vi "Parallel_FFTs.vi"(10 "SampleRate":dbl, 11 "Y":cdb[](array[numeric])) -> (2 "PeakValues":dbl[](array[numeric]), 3 "10 Hz FFTs":dbl[][](array[numeric]))   [LabVIEW 2018]
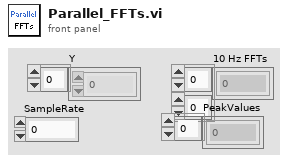
[diagram p1: front panel]
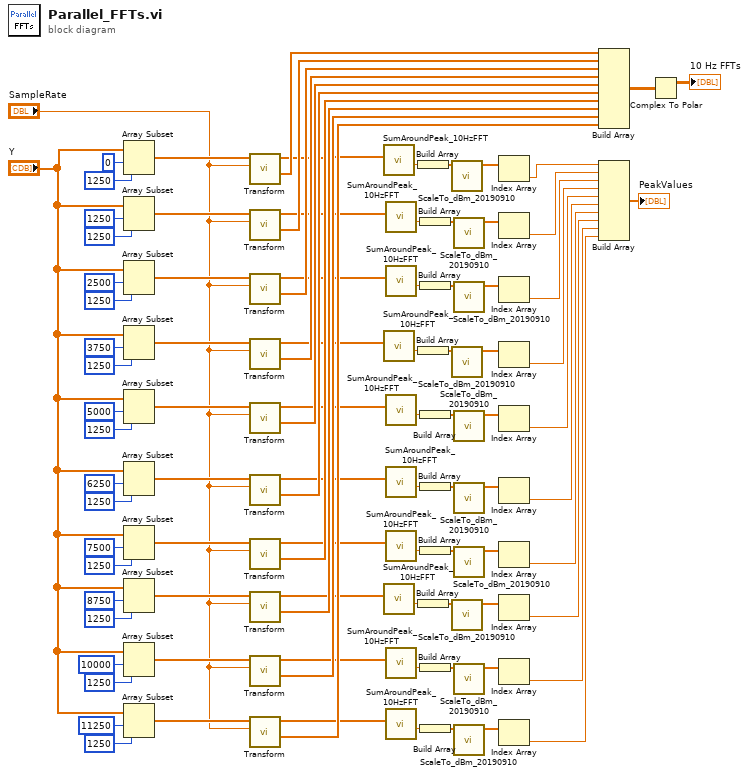
[diagram p0: block diagram]
diagram:
  n1 = Array Subset(array="Y", index=0, length=1250) -> (w76:cdb[])
  n2 = Array Subset(array="Y", index=1250, length=1250) -> (w77:cdb[])
  n3 = Array Subset(array="Y", index=2500, length=1250) -> (w78:cdb[])
  n4 = Array Subset(array="Y", index=3750, length=1250) -> (w79:cdb[])
  n5 = Array Subset(array="Y", index=5000, length=1250) -> (w80:cdb[])
  n6 = Array Subset(array="Y", index=6250, length=1250) -> (w81:cdb[])
  n7 = Array Subset(array="Y", index=7500, length=1250) -> (w82:cdb[])
  n8 = Array Subset(array="Y", index=8750, length=1250) -> (w83:cdb[])
  n9 = Array Subset(array="Y", index=10000, length=1250) -> (w84:cdb[])
  n10 = Array Subset(array="Y", index=11250, length=1250) -> (w85:cdb[])
  n11 = call "Transform.vi"("SampleRate"="SampleRate", "TimeDomainIn"=w76) -> ("Complex"=w61:cdb[], "AmplitudeSpectrum"=w44:dbl[])  [unwired: 4 in, 4 out]
  n12 = call "Transform.vi"("SampleRate"="SampleRate", "TimeDomainIn"=w77) -> ("Complex"=w60:cdb[], "AmplitudeSpectrum"=w49:dbl[])  [unwired: 4 in, 4 out]
  n13 = call "Transform.vi"("SampleRate"="SampleRate", "TimeDomainIn"=w78) -> ("Complex"=w59:cdb[], "AmplitudeSpectrum"=w41:dbl[])  [unwired: 4 in, 4 out]
  n14 = call "Transform.vi"("SampleRate"="SampleRate", "TimeDomainIn"=w79) -> ("Complex"=w58:cdb[], "AmplitudeSpectrum"=w32:dbl[])  [unwired: 4 in, 4 out]
  n15 = call "Transform.vi"("SampleRate"="SampleRate", "TimeDomainIn"=w80) -> ("Complex"=w57:cdb[], "AmplitudeSpectrum"=w33:dbl[])  [unwired: 4 in, 4 out]
  n16 = call "Transform.vi"("SampleRate"="SampleRate", "TimeDomainIn"=w81) -> ("Complex"=w56:cdb[], "AmplitudeSpectrum"=w34:dbl[])  [unwired: 4 in, 4 out]
  n17 = call "Transform.vi"("SampleRate"="SampleRate", "TimeDomainIn"=w82) -> ("Complex"=w55:cdb[], "AmplitudeSpectrum"=w23:dbl[])  [unwired: 4 in, 4 out]
  n18 = call "Transform.vi"("SampleRate"="SampleRate", "TimeDomainIn"=w83) -> ("Complex"=w54:cdb[], "AmplitudeSpectrum"=w22:dbl[])  [unwired: 4 in, 4 out]
  n19 = call "Transform.vi"("SampleRate"="SampleRate", "TimeDomainIn"=w84) -> ("Complex"=w53:cdb[], "AmplitudeSpectrum"=w21:dbl[])  [unwired: 4 in, 4 out]
  n20 = call "Transform.vi"("SampleRate"="SampleRate", "TimeDomainIn"=w85) -> ("Complex"=w52:cdb[], "AmplitudeSpectrum"=w20:dbl[])  [unwired: 4 in, 4 out]
  n21 = call "SumAroundPeak_10HzFFT.vi"("spectrum in"=w44) -> ("SumOfPeak"=w46:dbl)  [unwired: 8 in, 2 out]
  n22 = call "SumAroundPeak_10HzFFT.vi"("spectrum in"=w32) -> ("SumOfPeak"=w38:dbl)  [unwired: 8 in, 2 out]
  n23 = call "SumAroundPeak_10HzFFT.vi"("spectrum in"=w22) -> ("SumOfPeak"=w28:dbl)  [unwired: 8 in, 2 out]
  n24 = call "SumAroundPeak_10HzFFT.vi"("spectrum in"=w49) -> ("SumOfPeak"=w50:dbl)  [unwired: 8 in, 2 out]
  n25 = call "SumAroundPeak_10HzFFT.vi"("spectrum in"=w41) -> ("SumOfPeak"=w42:dbl)  [unwired: 8 in, 2 out]
  n26 = call "SumAroundPeak_10HzFFT.vi"("spectrum in"=w33) -> ("SumOfPeak"=w35:dbl)  [unwired: 8 in, 2 out]
  n27 = call "SumAroundPeak_10HzFFT.vi"("spectrum in"=w34) -> ("SumOfPeak"=w40:dbl)  [unwired: 8 in, 2 out]
  n28 = call "SumAroundPeak_10HzFFT.vi"("spectrum in"=w23) -> ("SumOfPeak"=w25:dbl)  [unwired: 8 in, 2 out]
  n29 = call "SumAroundPeak_10HzFFT.vi"("spectrum in"=w21) -> ("SumOfPeak"=w31:dbl)  [unwired: 8 in, 2 out]
  n30 = call "SumAroundPeak_10HzFFT.vi"("spectrum in"=w20) -> ("SumOfPeak"=w26:dbl)  [unwired: 8 in, 2 out]
  n31 = Build Array(w46) -> (w47:dbl[])
  n32 = Build Array(w38) -> (w37:dbl[])
  n33 = Build Array(w28) -> (w29:dbl[])
  n34 = Build Array(w50) -> (w48:dbl[])
  n35 = Build Array(w42) -> (w43:dbl[])
  n36 = Build Array(w35) -> (w36:dbl[])
  n37 = Build Array(w40) -> (w39:dbl[])
  n38 = Build Array(w25) -> (w24:dbl[])
  n39 = Build Array(w31) -> (w30:dbl[])
  n40 = Build Array(w26) -> (w27:dbl[])
  n41 = call "ScaleTo_dBm_20190910.vi"("Power Spectrum In (Volts)"=w47) -> ("P (dBm)"=w45:dbl[])  [unwired: 10 in]
  n42 = call "ScaleTo_dBm_20190910.vi"("Power Spectrum In (Volts)"=w37) -> ("P (dBm)"=w13:dbl[])  [unwired: 10 in]
  n43 = call "ScaleTo_dBm_20190910.vi"("Power Spectrum In (Volts)"=w29) -> ("P (dBm)"=w6:dbl[])  [unwired: 10 in]
  n44 = call "ScaleTo_dBm_20190910.vi"("Power Spectrum In (Volts)"=w48) -> ("P (dBm)"=w17:dbl[])  [unwired: 10 in]
  n45 = call "ScaleTo_dBm_20190910.vi"("Power Spectrum In (Volts)"=w43) -> ("P (dBm)"=w16:dbl[])  [unwired: 10 in]
  n46 = call "ScaleTo_dBm_20190910.vi"("Power Spectrum In (Volts)"=w36) -> ("P (dBm)"=w12:dbl[])  [unwired: 10 in]
  n47 = call "ScaleTo_dBm_20190910.vi"("Power Spectrum In (Volts)"=w39) -> ("P (dBm)"=w10:dbl[])  [unwired: 10 in]
  n48 = call "ScaleTo_dBm_20190910.vi"("Power Spectrum In (Volts)"=w24) -> ("P (dBm)"=w8:dbl[])  [unwired: 10 in]
  n49 = call "ScaleTo_dBm_20190910.vi"("Power Spectrum In (Volts)"=w30) -> ("P (dBm)"=w4:dbl[])  [unwired: 10 in]
  n50 = call "ScaleTo_dBm_20190910.vi"("Power Spectrum In (Volts)"=w27) -> ("P (dBm)"=w2:dbl[])  [unwired: 10 in]
  n51 = Index Array(array=w45) -> (element=w19:dbl)  [unwired: 1 in]
  n52 = Index Array(array=w17) -> (element=w18:dbl)  [unwired: 1 in]
  n53 = Index Array(array=w16) -> (element=w15:dbl)  [unwired: 1 in]
  n54 = Index Array(array=w13) -> (element=w14:dbl)  [unwired: 1 in]
  n55 = Index Array(array=w12) -> (element=w11:dbl)  [unwired: 1 in]
  n56 = Index Array(array=w10) -> (element=w9:dbl)  [unwired: 1 in]
  n57 = Index Array(array=w8) -> (element=w7:dbl)  [unwired: 1 in]
  n58 = Index Array(array=w6) -> (element=w5:dbl)  [unwired: 1 in]
  n59 = Index Array(array=w4) -> (element=w3:dbl)  [unwired: 1 in]
  n60 = Index Array(array=w2) -> (element=w1:dbl)  [unwired: 1 in]
  n61 = Build Array(w61, w60, w59, w58, w57, w56, w55, w54, w53, w52) -> (w62:cdb[][])
  n62 = Build Array(w19, w18, w15, w14, w11, w9, w7, w5, w3, w1) -> (→"PeakValues":dbl[])
  n63 = Complex To Polar(r * e^(i*theta)=w62) -> (r=→"10 Hz FFTs":dbl[][])  [unwired: 1 out]
